vi "XCP DAQ Read Waveform.vi"(8 "error in (no error)":errorcluster, 9 "timeout (1s)":dbl=1.0 format="%#_13g", 10 "Number of Sample":i32, 11 "DAQList in":refnum<class "DAQList.lvclass">) -> (0 "error out":errorcluster, 1 "Data":waveform(dbl)[](array[waveform]), 2 "Number of Sample Returned":i32, 3 "DAQList out":refnum<class "DAQList.lvclass">)   [LabVIEW 2019, in "XCP_DaqDtoId.lvlib" / "DAQList.lvclass"]
uses:
  DAQList.lvclass
  DAQList.lvclass/DAQList.ctl
  XnetRead/SubVI_MergeData2.vi
  XcpCommand/SendCommands.vi
  XcpCommand/FilterCommands.vi
  DatabaseGeneration/CreateCluster.vi
  DatabaseGeneration/CreateFrames.vi
  XnetRead/InitXnet.vi
  DatabaseGeneration/CreateSignals_SingleByte.vi
  DatabaseGeneration/SubVI_FilterDaqProcessorInfo.vi
  DatabaseGeneration/SubVI_FilterDaqResolutionInfo.vi
  XnetRead/InitMeaSplitInfo2.vi
  DatabaseGeneration/SubVI_SetMeasProp.vi
  DatabaseGeneration/SubVI_ProcessMaxOdtEntrySize.vi
  <vilib>/xnet/xnet.llb/XNET Create Session.vi
  <vilib>/xnet/xnet.llb/XNET Create Session (Frame Input Stream).vi
  <vilib>/xnet/xnet.llb/XNET Start.vi
  <vilib>/ECUMC/ECUMC.llb/MC DAQ List Initialize.vi
  <vilib>/ECUMC/ECUMC.llb/MC ECU Connect.vi
  <vilib>/ECUMC/ECUMC.llb/MC DAQ Start Stop.vi
  <vilib>/xnet/xnet.llb/XNET Read (Frame CAN).vi
  <vilib>/xnet/xnet.llb/XNET Clear.vi
  <vilib>/ECUMC/ECUMC.llb/MC Get Property.vi
  <vilib>/ECUMC/ECUMC.llb/MC Get Prop XCP CRO Id.vi
  <vilib>/ECUMC/ECUMC.llb/MC Get Prop XCP DTO Id.vi
  <vilib>/ECUMC/ECUMC.llb/MC Get Prop XCP CAN IO Mode.vi
  <vilib>/ECUMC/ECUMC.llb/MC Get Prop XCP Baud Rate 64.vi
  <vilib>/ECUMC/ECUMC.llb/MC Get Prop XCP FD Baud Rate 64.vi
  <vilib>/xnet/xnet.llb/XNET Database Create Object.vi
  <vilib>/xnet/xnet.llb/XNET Database Create (Cluster).vi
  <vilib>/Utility/error.llb/Error Cluster From Error Code.vi
  <vilib>/xnet/xnet.llb/XNET Database Create (Frame).vi
  <vilib>/Utility/file.llb/Application Directory.vi
  <vilib>/xnet/xnet.llb/XNET Database Save.vi
  DatabaseGeneration/CreateSignals.vi
  <vilib>/ECUMC/ECUMC.llb/MC Get Prop Meas Address.vi
  <vilib>/xnet/xnet.llb/XNET Database Create (Signal).vi
  <vilib>/xnet/xnet.llb/XNET Database Create (Subframe).vi
  <vilib>/ECUMC/ECUMC.llb/MC Get Prop Meas Data Type.vi
  <vilib>/xnet/xnet.llb/XNET Database Create (Dynamic Signal).vi
  <vilib>/ECUMC/ECUMC.llb/MC Get Prop Meas Comment.vi
  <vilib>/ECUMC/ECUMC.llb/MC Get Prop Meas Scaling Offset.vi
  <vilib>/ECUMC/ECUMC.llb/MC Get Prop Meas Scaling Factor.vi
  <vilib>/ECUMC/ECUMC.llb/MC Get Prop Meas Minimum.vi
  <vilib>/ECUMC/ECUMC.llb/MC Get Prop Meas Maximum.vi
  <vilib>/ECUMC/ECUMC.llb/MC Get Prop Meas Byte Order.vi
  <vilib>/ECUMC/ECUMC.llb/MC Get Prop Meas Unit.vi
  <vilib>/xnet/xnet.llb/XNET Create Session (Signal Input Waveform).vi
  TypeDef/Global.vi
  <vilib>/xnet/xnet.llb/XNET Read (Signal Waveform) .vi
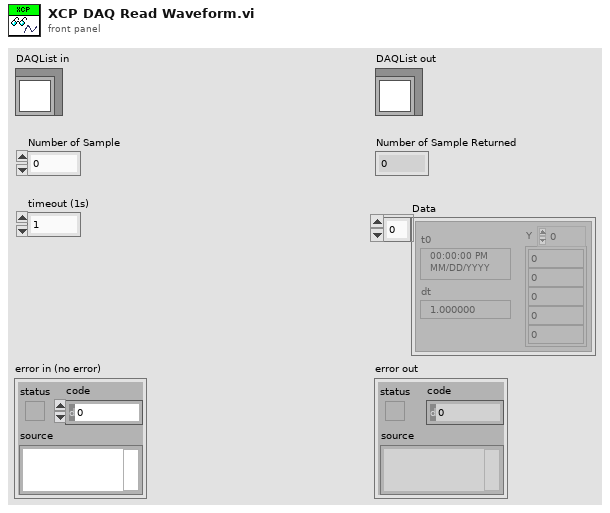
[diagram p1: front panel]
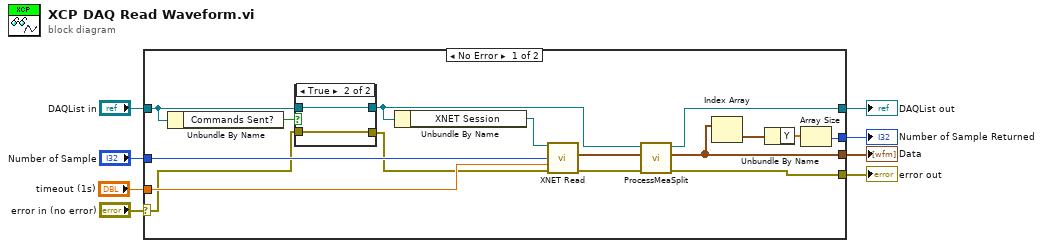
[diagram p0: block diagram]
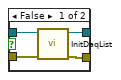
[diagram p2: hidden frame]
diagram:
  n1 = case shown="No Error" "error in (no error)" {
    selector: "error in (no error)" -> [w10 w32]
    tunnel: [w20 w32] -> w7
    tunnel: [w22 w31] -> w5
    tunnel: "DAQList in" -> [w11 w31]
    tunnel: "Number of Sample" -> [w23 _]
    tunnel: [w14 _] -> w3
    tunnel: "timeout (1s)" -> [w17 _]
    tunnel: [w15 _] -> w1
    frame No Error {
      n2 = Unbundle By Name(w11) -> ("Commands Sent?"=w13:bool)
      n3 = case shown="True" w13 {
        tunnel: w11 -> [w28 w30]
        tunnel: [w27 w30] -> w12
        tunnel: w10 -> [w26 w29]
        tunnel: [w25 w29] -> w9
        frame False {
          n4 = call "InitDaqList.vi"("error in (no error)"=w26, "DAQList in"=w28) -> ("error out"=w25:errorcluster, "DAQList out"=w27:refnum<class "DAQList.lvclass">)  [unwired: 8 in]
        }
        frame True {
        }
      }
      n5 = Unbundle By Name(w12) -> ("XNET Session"=w24:refnum<k21>)
      n6 = call-poly <vilib>:"XNET Read.vi"("session in"=w24, "number to read (-1)"=w23, "timeout (0)"=w17, "error in (no error)"=w9) -> ("data"=w19:waveform(dbl)[], "error out"=w21:errorcluster)  [unwired: 10 out]
      n7 = call "ProcessMeaSplit.vi"("error in (no error)"=w21, "Data In"=w19, "DAQList in"=w12) -> ("error out"=w20:errorcluster, "Data Out"=w14:waveform(dbl)[], "DAQList out"=w22:refnum<class "DAQList.lvclass">)  [unwired: 6 in]
      n8 = Index Array(array=w14) -> (element=w18:waveform(dbl))  [unwired: 1 in]
      n9 = Unbundle By Name(w18) -> ("Y"=w16:dbl[])
      n10 = Array Size(array=w16) -> (size(s)=w15:i32)
    }
    frame Error {
    }
  }
  "error out" <- w7
  "DAQList out" <- w5
  "Data" <- w3
  "Number of Sample Returned" <- w1
